vi "DHE_LoadDHEModule.vi"(8 "error in (no error)":errorcluster, 10 "ModuleName":string, 11 "modpath":path) -> (0 "error out":errorcluster)   [LabVIEW 2016]
panel:
  in  "type specifier VI Refnum (for type only)":refnum<vi>
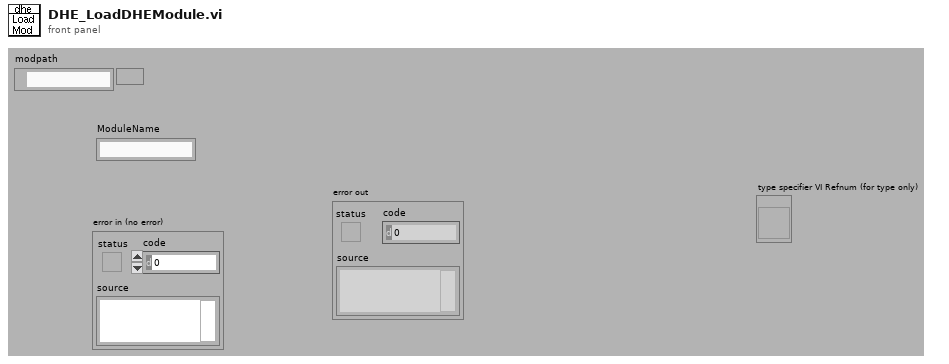
[diagram p1: front panel]
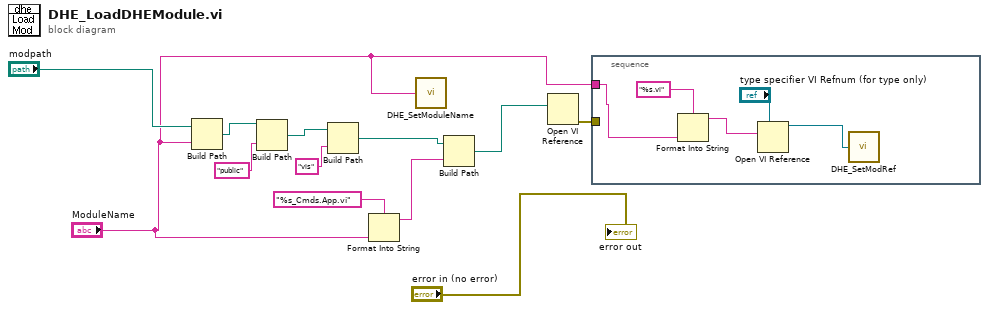
[diagram p0: block diagram]
diagram:
  n1 = Build Path(base path="modpath", name or relative path="ModuleName") -> (appended path=w12:path)
  n2 = Build Path(base path=w12, name or relative path="public") -> (appended path=w10:path)
  n3 = Build Path(base path=w10, name or relative path="vis") -> (appended path=w7:path)
  n4 = Format Into String(format string="%s_Cmds.App.vi", "ModuleName") -> (resulting string=w6:string)  [unwired: 2 in, 1 out]
  n5 = call "DHE_SetModuleName.vi"("DHE_ModuleName"="ModuleName") -> ()  [unwired: 9 out]
  n6 = Build Path(base path=w7, name or relative path=w6) -> (appended path=w5:path)
  n7 = Open VI Reference(vi path=w5) -> (error out=w3:errorcluster)  [unwired: 1 in, 5 out]
  n8 = stacked-sequence {
    tunnel: w3 -> [_]
    tunnel: "ModuleName" -> [w13]
    frame #0 {
      n9 = Format Into String(format string="%s.vi", w13) -> (resulting string=w15:string)  [unwired: 2 in, 1 out]
      n10 = Open VI Reference(type specifier VI Refnum (for type only)="type specifier VI Refnum (for type only)", vi path=w15) -> (vi reference=w14:refnum<vi>)  [unwired: 1 in, 4 out]
      n11 = call "DHE_SetModRef.vi"("DHE_ModRef"=w14) -> ()  [unwired: 9 out]
    }
  }
  "error out" <- "error in (no error)"
